vi "Digital Write N Chans.vi"(8 "Error In":errorcluster, 9 "Values":bool[](array[boolean]), 10 "DO Channels":u8[](array[numeric]), 11 "LINX Resource":T1) -> (0 "Error Out":errorcluster, 3 "LINX Resource":T1)   [LabVIEW 2013, in "LVH-LINX.lvlib"]
doc: "Write values to the specified digital output channels."
uses:
  <vilib>/LabVIEW Hacker/LINX/LVH-LINX.lvlib
  <vilib>/LabVIEW Hacker/LINX/Private/Type Defs/LINX Ref.ctl
  <vilib>/LabVIEW Hacker/LINX/Private/Type Defs/Platform.ctl
  <vilib>/LabVIEW Hacker/LINX/Private/Type Defs/Interface.ctl
  <vilib>/LabVIEW Hacker/LINX/Private/Device/Type Defs/LINX Device Config.ctl
  <vilib>/LabVIEW Hacker/LINX/Private/Device/Type Defs/TCP Config.ctl
  <vilib>/LabVIEW Hacker/LINX/Private/Type Defs/Device Family.ctl
  <vilib>/LabVIEW Hacker/LINX/Private/Type Defs/Peripheral.ctl
  <vilib>/LabVIEW Hacker/LINX/Private/Device/Device.lvlib
  <vilib>/LabVIEW Hacker/LINX/Private/myRIO/myRIO.lvlib
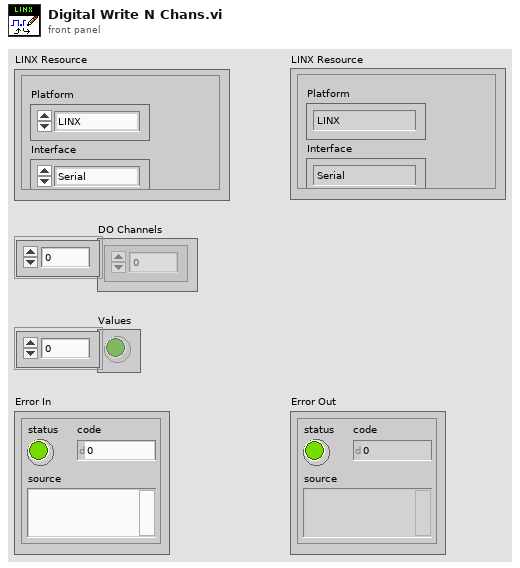
[diagram p1: front panel]
types:
  T1 = typedef "LVH-LINX.lvlib/LINX Ref.ctl" = cluster{"Platform":T2, "Interface":T3, "LINX Device Config":T4}
  T2 = typedef "LVH-LINX.lvlib/Platform.ctl" = enum16{"LINX", "myRIO"}
  T3 = typedef "LVH-LINX.lvlib/Interface.ctl" = enum16{"Serial", "TCP"}
  T4 = typedef "LVH-LINX.lvlib/Device.lvlib/LINX Device Config.ctl" = cluster{"Interface":T3, "COM Port":refnum<visa-resource-name>, "TCP Configuration":T5, "Device Family":T6, "Device ID":u8, "Device Name":string, "TCP Ref":refnum<k5>}
  T5 = typedef "LVH-LINX.lvlib/Device.lvlib/TCP Config.ctl" = cluster{"IP Address":string, "Port":u16}
  T6 = typedef "LVH-LINX.lvlib/Device Family.ctl" = enum8{"National Instruments", "Digilent", "Arduino"}
  T7 = typedef "LVH-LINX.lvlib/Peripheral.ctl" = enum8{"DI", "DO", "AI", "AO", "PWM", "QE", "UART", "I2C", "SPI", "CAN"}
  T8 = typedef "DIO.lvlib/DIO Reference.ctl" = cluster{"myRIO Reference":T9, "DIO Channels List":T13}
  T9 = typedef "myRIO Generic Hardware Reference.ctl" = cluster{"myRIO Model":T10, "myRIO Hardware Reference":T11}
  T10 = typedef "Hardware Version Enum.ctl" = enum16{"Unknown", "myRIO-1900", "myRIO-1950"}
  T11 = typedef "myRIO v1.0 Reference.ctl" = cluster{"Generic FPGA Reference":T12, "Allow multiple opens":bool}
  T12 = typedef "Generic FPGA Reference.ctl" = refnum<k20>
  T13 = typedef "DIO Channels List.ctl" = T14[]
  T14 = typedef "DIO Channels Enum.ctl" = enum16{"Not Connected", "C/DIO0", "C/DIO1", "C/DIO2", "C/DIO3", "C/DIO4", "C/DIO5", "C/DIO6", "C/DIO7", "A/DIO0", "A/DIO1", "A/DIO2", "A/DIO3", "A/DIO4", "A/DIO5", "A/DIO6", "A/DIO7", "A/DIO8", "A/DIO9", "A/DIO10", "A/DIO11", "A/DIO12", "A/DIO13", "A/DIO14", "A/DIO15", "B/DIO0", "B/DIO1", "B/DIO2", "B/DIO3", "B/DIO4", "B/DIO5", "B/DIO6", "B/DIO7", "B/DIO8", "B/DIO9", "B/DIO10", "B/DIO11", "B/DIO12", "B/DIO13", "B/DIO14", "B/DIO15", "LED0", "LED1", "LED2", "LED3", "Button0"}
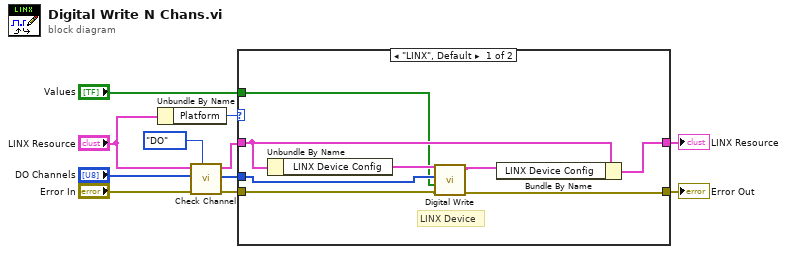
[diagram p0: block diagram]
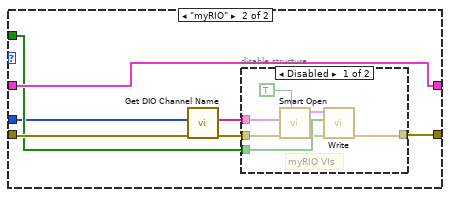
[diagram p2: hidden frame]
diagram:
  n1 = Unbundle By Name("LINX Resource") -> ("Platform"=w11:T2)
  n2 = call <vilib>:"Check Channel.vi"("Peripheral"=Peripheral."DO", "Error In"="Error In", "Channels"="DO Channels", "LINX Resource"="LINX Resource") -> ("Error Out"=w4:errorcluster, "Channels"=w3:u8[], "LINX Resource"=w6:T1)  [unwired: 5 in]
  n3 = case shown="\"LINX\", Default" w11 {
    tunnel: w4 -> [w14 w25]
    tunnel: w6 -> [w19 w26]
    tunnel: [w17 w22] -> w10
    tunnel: [w18 w26] -> w9
    tunnel: "Values" -> [w12 w21]
    tunnel: w3 -> [w13 w20]
    frame "LINX", Default {
      # "LINX Device"
      n4 = Unbundle By Name(w19) -> ("LINX Device Config"=w15:T4)
      n5 = call <vilib>:"Digital Write.vi"("Error In"=w14, "Values"=w12, "Channels"=w13, "LINX Device Config"=w15) -> ("Error Out"=w17:errorcluster, "LINX Device Config"=w16:T4)  [unwired: 6 in]
      n6 = Bundle By Name(cluster=w19, "LINX Device Config"=w16) -> (w18:T1)
    }
    frame "myRIO" {
      n7 = call <vilib>:"Get DIO Channel Name.vi"("Error In"=w25, "DIO Channel Nums"=w20) -> ("Error Out"=w23:errorcluster, "DIO Channels"=w24:string[])  [unwired: 8 in]
      n8 = disable-structure shown="Disabled" {
        disable-tunnel: w24 -> [w29 _]
        disable-tunnel: w23 -> [w30 w34]
        disable-tunnel: w21 -> [w33 _]
        disable-tunnel: [w32 w34] -> w22
        frame Disabled {
          # "myRIO VIs"
          n9 = call <vilib>:"Smart Open.vi"("Allow multiple opens?"=TRUE, "error in (no error)"=w30, "Channel Names"=w29) -> ("error out"=w31:errorcluster, "DIO Ref Out"=w28:T8)  [unwired: 7 in]
          n10 = call <vilib>:"Write.vi"("error in (no error)"=w31, "Values"=w33, "DIO Ref In"=w28) -> ("error out"=w32:errorcluster)  [unwired: 6 in, 1 out]
        }
        frame Enabled {
          # "myRIO Support Disabled"
        }
      }
    }
  }
  "Error Out" <- w10
  "LINX Resource" <- w9
